vi "ball.vi"(7 "Numeric":i8, 8 "error in (no error)":errorcluster, 11 "KNR in":T1) -> (0 "error out":errorcluster, 3 "KNR out":T1, 4 "ball offset":i32)   [LabVIEW 2013]
uses:
  <userlib>/KNR OS 3.0 LabVIEW Toolkit/Type Definition/KNR3 Reference.ctl
  <userlib>/_FPGA Interface Advanced Tools/FPGA Interface Base/FPGA Interface Base.lvclass
  <userlib>/KNR OS 3.0 LabVIEW Toolkit/Type Definition/Resource.ctl
  Global 1.vi
panel:
  in  "STOP 2":bool
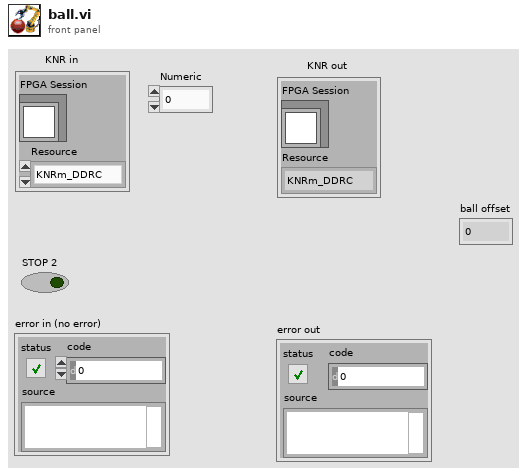
[diagram p1: front panel]
types:
  T1 = typedef "KNR3 Reference.ctl" = cluster{"FPGA Session":refnum<class "FPGA Interface Base.lvclass">, "Resource":T2}
  T2 = typedef "Resource.ctl" = enum16{"KNRm_DDRC", "KNRm_DDDD", "KNRm_DDDR", "KNRm_DDDC", "KNR"}
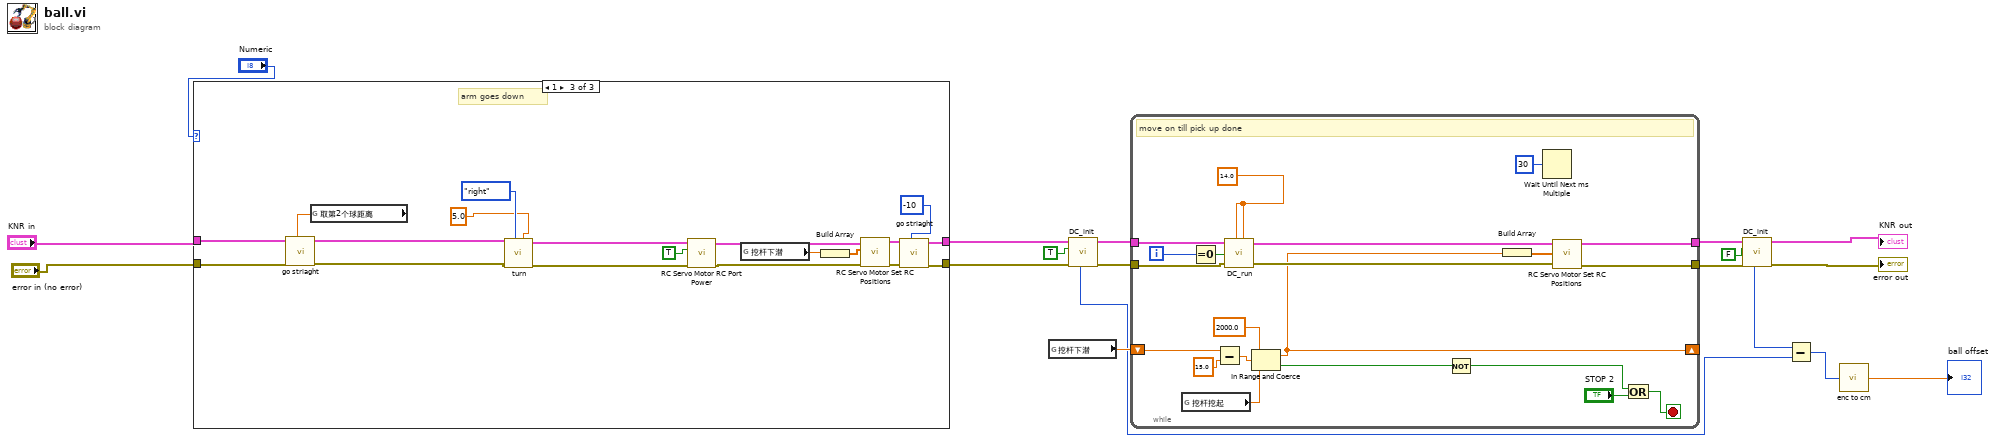
[diagram p0: block diagram]
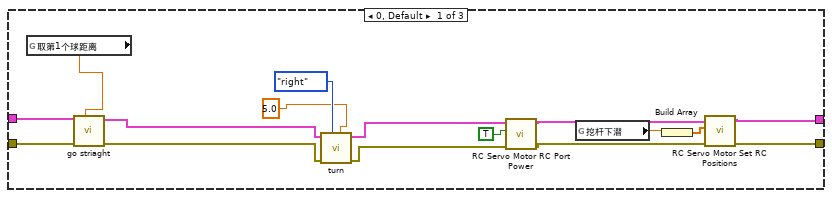
[diagram p2: hidden frame]
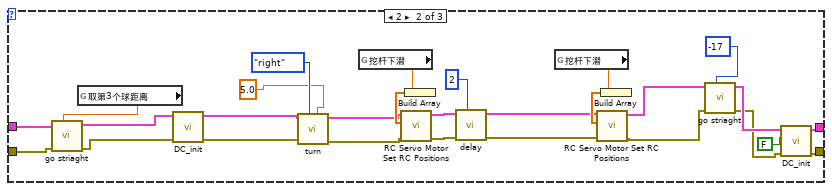
[diagram p3: hidden frame]
diagram:
  n1 = case shown="1" "Numeric" {
    tunnel: "KNR in" -> [w25 w42 w71]
    tunnel: "error in (no error)" -> [w34 w41 w70]
    tunnel: [w29 w61 w79] -> w8
    tunnel: [w28 w60 w78] -> w7
    frame 0, Default {
      n2 = global read "Global 1.vi" "取第1个球距离"() -> (w33:dbl)
      n3 = call "go striaght.vi"("距离"=w33, "error in (no error)"=w34, "KNR in"=w25) -> ("error out"=w20:errorcluster, "KNR out"=w22:T1)  [unwired: 7 in]
      n4 = call "turn.vi"("Angle"=5.0, "side"=enum16{"right", "left"}."right", "error in (no error)"=w20, "KNR in"=w22) -> ("error out"=w19:errorcluster, "KNR out"=w21:T1)  [unwired: 6 in]
      n5 = call <userlib>:"RC Servo Motor RC Port Power.vi"("error in (no error)"=w19, "RC Power(F)"=TRUE, "KNR in"=w21) -> ("error out"=w26:errorcluster, "KNR out"=w27:T1)  [unwired: 7 in]
      n6 = global read "Global 1.vi" "挖杆下潜"() -> (w30:dbl)
      n7 = Build Array(w30) -> (w31:dbl[])
      n8 = call <userlib>:"RC Servo Motor Set RC Positions.vi"("error in (no error)"=w26, "RC Pulse Width (1500 uS)"=w31, "KNR in"=w27) -> ("error out"=w28:errorcluster, "KNR out"=w29:T1)  [unwired: 7 in]
    }
    frame 2 {
      n9 = global read "Global 1.vi" "取第3个球距离"() -> (w45:dbl)
      n10 = call "go striaght.vi"("距离"=w45, "error in (no error)"=w41, "KNR in"=w42) -> ("error out"=w43:errorcluster, "KNR out"=w44:T1)  [unwired: 7 in]
      n11 = call "DC_init.vi"("error in (no error)"=w43, "KNR in"=w44) -> ("error out"=w37:errorcluster, "KNR out"=w38:T1)  [unwired: 6 in, 2 out]
      n12 = call "turn.vi"("Angle"=5.0, "side"=enum16{"right", "left"}."right", "error in (no error)"=w37, "KNR in"=w38) -> ("error out"=w35:errorcluster, "KNR out"=w36:T1)  [unwired: 6 in]
      n13 = global read "Global 1.vi" "挖杆下潜"() -> (w51:dbl)
      n14 = Build Array(w51) -> (w52:dbl[])
      n15 = call <userlib>:"RC Servo Motor Set RC Positions.vi"("error in (no error)"=w35, "RC Pulse Width (1500 uS)"=w52, "KNR in"=w36) -> ("error out"=w49:errorcluster, "KNR out"=w50:T1)  [unwired: 7 in]
      n16 = call "delay.vi"("Numeric"=2, "error in (no error)"=w49, "KNR in"=w50) -> ("error out"=w47:errorcluster, "KNR out"=w48:T1)  [unwired: 7 in]
      n17 = global read "Global 1.vi" "挖杆下潜"() -> (w55:dbl)
      n18 = Build Array(w55) -> (w56:dbl[])
      n19 = call <userlib>:"RC Servo Motor Set RC Positions.vi"("error in (no error)"=w47, "RC Pulse Width (1500 uS)"=w56, "KNR in"=w48) -> ("error out"=w53:errorcluster, "KNR out"=w54:T1)  [unwired: 7 in]
      n20 = call "go striaght.vi"("距离"=-17 ("DST"), "error in (no error)"=w53, "KNR in"=w54) -> ("error out"=w57:errorcluster, "KNR out"=w58:T1)  [unwired: 7 in]
      n21 = call "DC_init.vi"("error in (no error)"=w57, "Enable Motor(T)"=FALSE, "KNR in"=w58) -> ("error out"=w60:errorcluster, "KNR out"=w61:T1)  [unwired: 5 in, 2 out]
    }
    frame 1 {
      # "arm goes down"
      n22 = global read "Global 1.vi" "取第2个球距离"() -> (w69:dbl)
      n23 = call "go striaght.vi"("距离"=w69, "error in (no error)"=w70, "KNR in"=w71) -> ("error out"=w63:errorcluster, "KNR out"=w66:T1)  [unwired: 7 in]
      n24 = call "turn.vi"("Angle"=5.0, "side"=enum16{"right", "left"}."right", "error in (no error)"=w63, "KNR in"=w66) -> ("error out"=w64:errorcluster, "KNR out"=w65:T1)  [unwired: 6 in]
      n25 = call <userlib>:"RC Servo Motor RC Port Power.vi"("error in (no error)"=w64, "RC Power(F)"=TRUE, "KNR in"=w65) -> ("error out"=w75:errorcluster, "KNR out"=w76:T1)  [unwired: 7 in]
      n26 = global read "Global 1.vi" "挖杆下潜"() -> (w72:dbl)
      n27 = Build Array(w72) -> (w77:dbl[])
      n28 = call <userlib>:"RC Servo Motor Set RC Positions.vi"("error in (no error)"=w75, "RC Pulse Width (1500 uS)"=w77, "KNR in"=w76) -> ("error out"=w73:errorcluster, "KNR out"=w74:T1)  [unwired: 7 in]
      n29 = call "go striaght.vi"("距离"=-10 ("DST"), "error in (no error)"=w73, "KNR in"=w74) -> ("error out"=w78:errorcluster, "KNR out"=w79:T1)  [unwired: 7 in]
    }
  }
  n30 = global read "Global 1.vi" "挖杆下潜"() -> (w10:dbl)
  n31 = call "DC_init.vi"("error in (no error)"=w7, "Enable Motor(T)"=TRUE, "KNR in"=w8) -> ("error out"=w9:errorcluster, "KNR out"=w11:T1, "output\nPosition_1"=w5:i32)  [unwired: 5 in, 1 out]
  n32 = while {
    tunnel: w11 -> [w91]
    tunnel: w9 -> [w89]
    tunnel: [w93] -> w17
    tunnel: [w92] -> w16
    shift-right: [w87] -> _
    shift-left: w10 -> [w97]
    i -> [w100]
    stop <- w102 stop-if-true
    w82 = 14.0
    # "move on till pick up done"
    n33 = global read "Global 1.vi" "挖杆挖起"() -> (w85:dbl)
    n34 = Equal To 0?(x=w100) -> (x = 0?=w86:bool)
    n35 = Subtract(x=w97, y=15.0) -> (x-y=w95:dbl)
    n36 = call "DC_run.vi"("KNR in"=w91, "speed_1"=w82, "reinitialize? (F)"=w86, "error in (no error)"=w89, "speed_2"=w82) -> ("KNR out"=w90:T1, "error out"=w88:errorcluster)  [unwired: 1 in, 2 out]
    n37 = In Range and Coerce(upper limit=2000.0, x=w95, lower limit=w85) -> (coerced(x)=w87:dbl, In Range?=w84:bool)
    n38 = Not(x=w84) -> (.not. x?=w83:bool)
    n39 = Build Array(w87) -> (w98:dbl[])
    n40 = Wait Until Next ms Multiple(millisecond multiple=u32 30) -> ()  [unwired: 1 out]
    n41 = call <userlib>:"RC Servo Motor Set RC Positions.vi"("error in (no error)"=w88, "RC Pulse Width (1500 uS)"=w98, "KNR in"=w90) -> ("error out"=w92:errorcluster, "KNR out"=w93:T1)  [unwired: 7 in]
    n42 = Or(x=w83, y="STOP 2") -> (x .or. y?=w102:bool)
  }
  n43 = call "DC_init.vi"("error in (no error)"=w16, "Enable Motor(T)"=FALSE, "KNR in"=w17) -> ("error out"=→"error out":errorcluster, "KNR out"=→"KNR out":T1, "output\nPosition_1"=w6:i32)  [unwired: 5 in, 1 out]
  n44 = Subtract(x=w6, y=w5) -> (x-y=w4:i32)
  n45 = call "enc to cm.vi"("E"=w4) -> ("CM"=→"ball offset":dbl)  [unwired: 1 in]
